vi "map_trap_switch.vi"() -> ()   [LabVIEW 2015]
panel:
  in  "KILL":bool
  in  "PAUSE":bool
  in  "RESUME":bool
  in  "QUIT":bool
  in  "up done":bool
  in  "z up":bool
  in  "Done":bool
  in  "z piastra 2":bool
  in  "z piastra":bool
  in  "y piastra":bool
  in  "x piastra":bool
  in  "goto y pos":bool
  in  "goto x pos":bool
  in  "Panello o piastre?":bool
  in  "End":bool
  in  "zero z - end":bool
  in  "zero x - end":bool
  in  "zero y - end":bool
  in  "goto z pos":bool
  in  "positioning done":bool
  out "output":string
  out "command":string
  in  "zero done":bool
  in  "zero z":bool
  in  "zero x":bool
  in  "zero y":bool
  # "Comandi di emergenza"
  # "Mappatura a trapezio \nper il pannello e le piastre"
  # "In alto: TRUE ---> Panello"
  # "In basso: FALSE ---> Piastre"
  # "Posiziono in zero"
  # "Vado sulla piastra \ne azzero"
  # "Alzo il comparatore"
  # "Vado in posizione"
  # "Ritorno a zero"
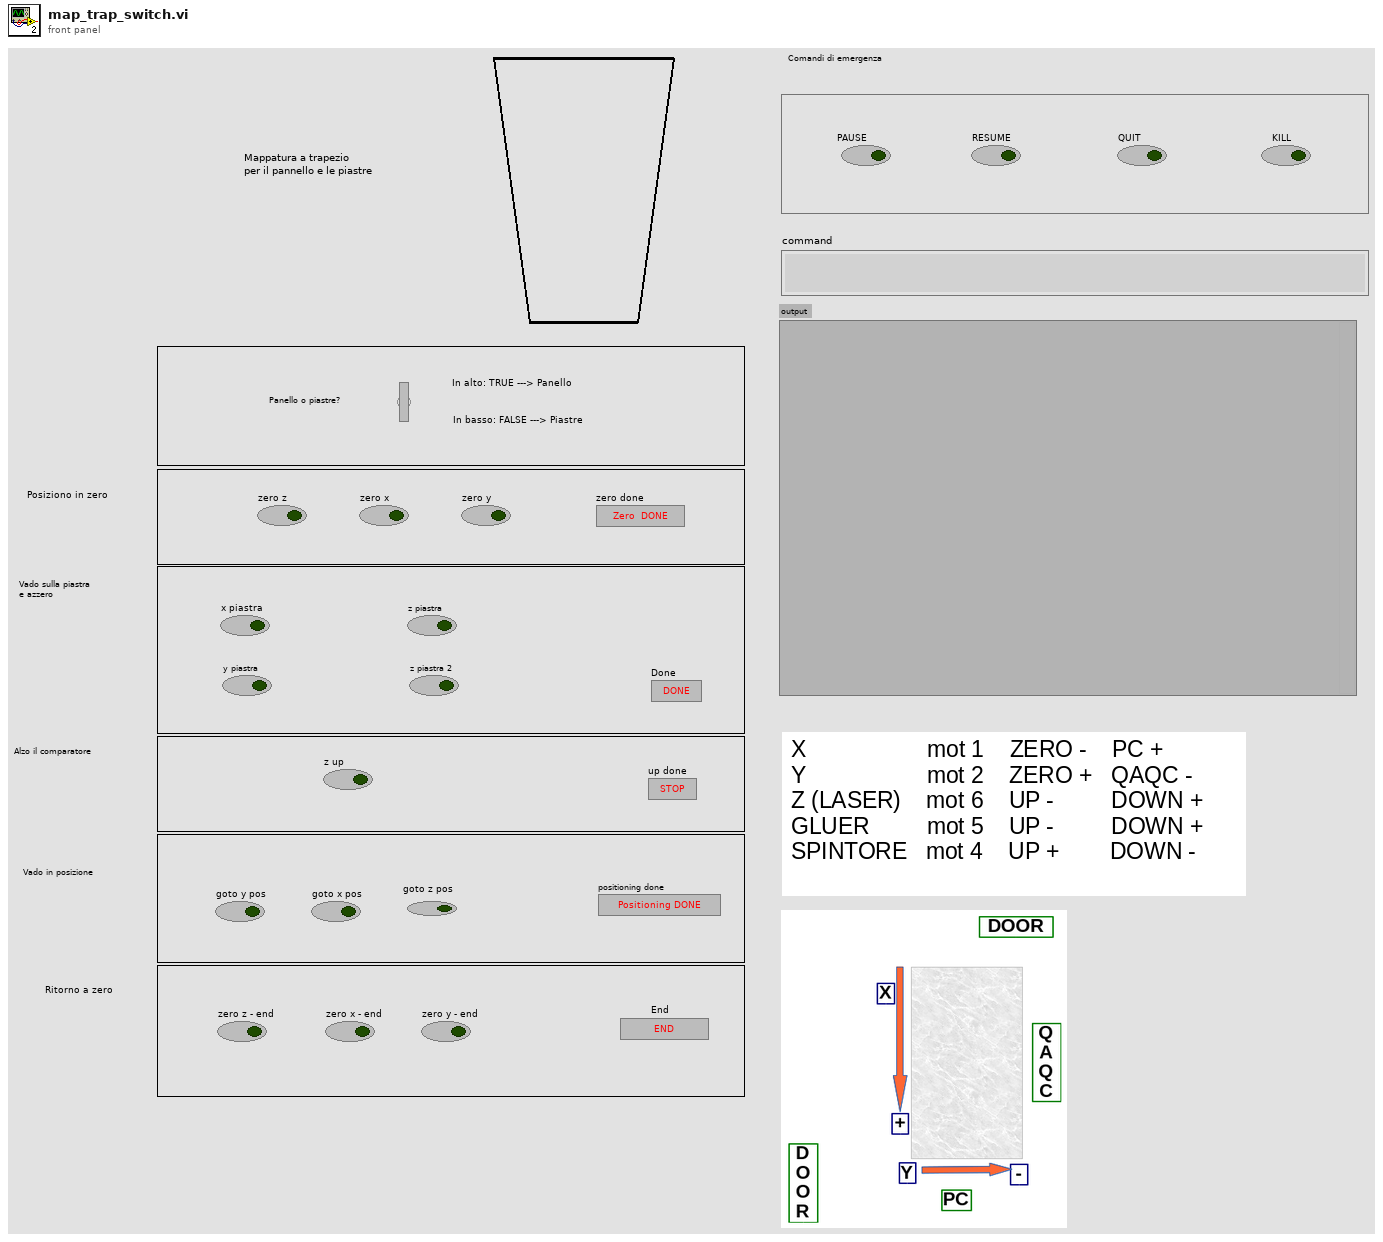
[diagram p1: front panel]
types:
  T1 = enum8{"Enabled", "Disabled", "Disabled and Grayed Out"}
  T2 = enum16{"open", "replace", "create", "open or create", "replace or create", "replace or create with confirmation"}
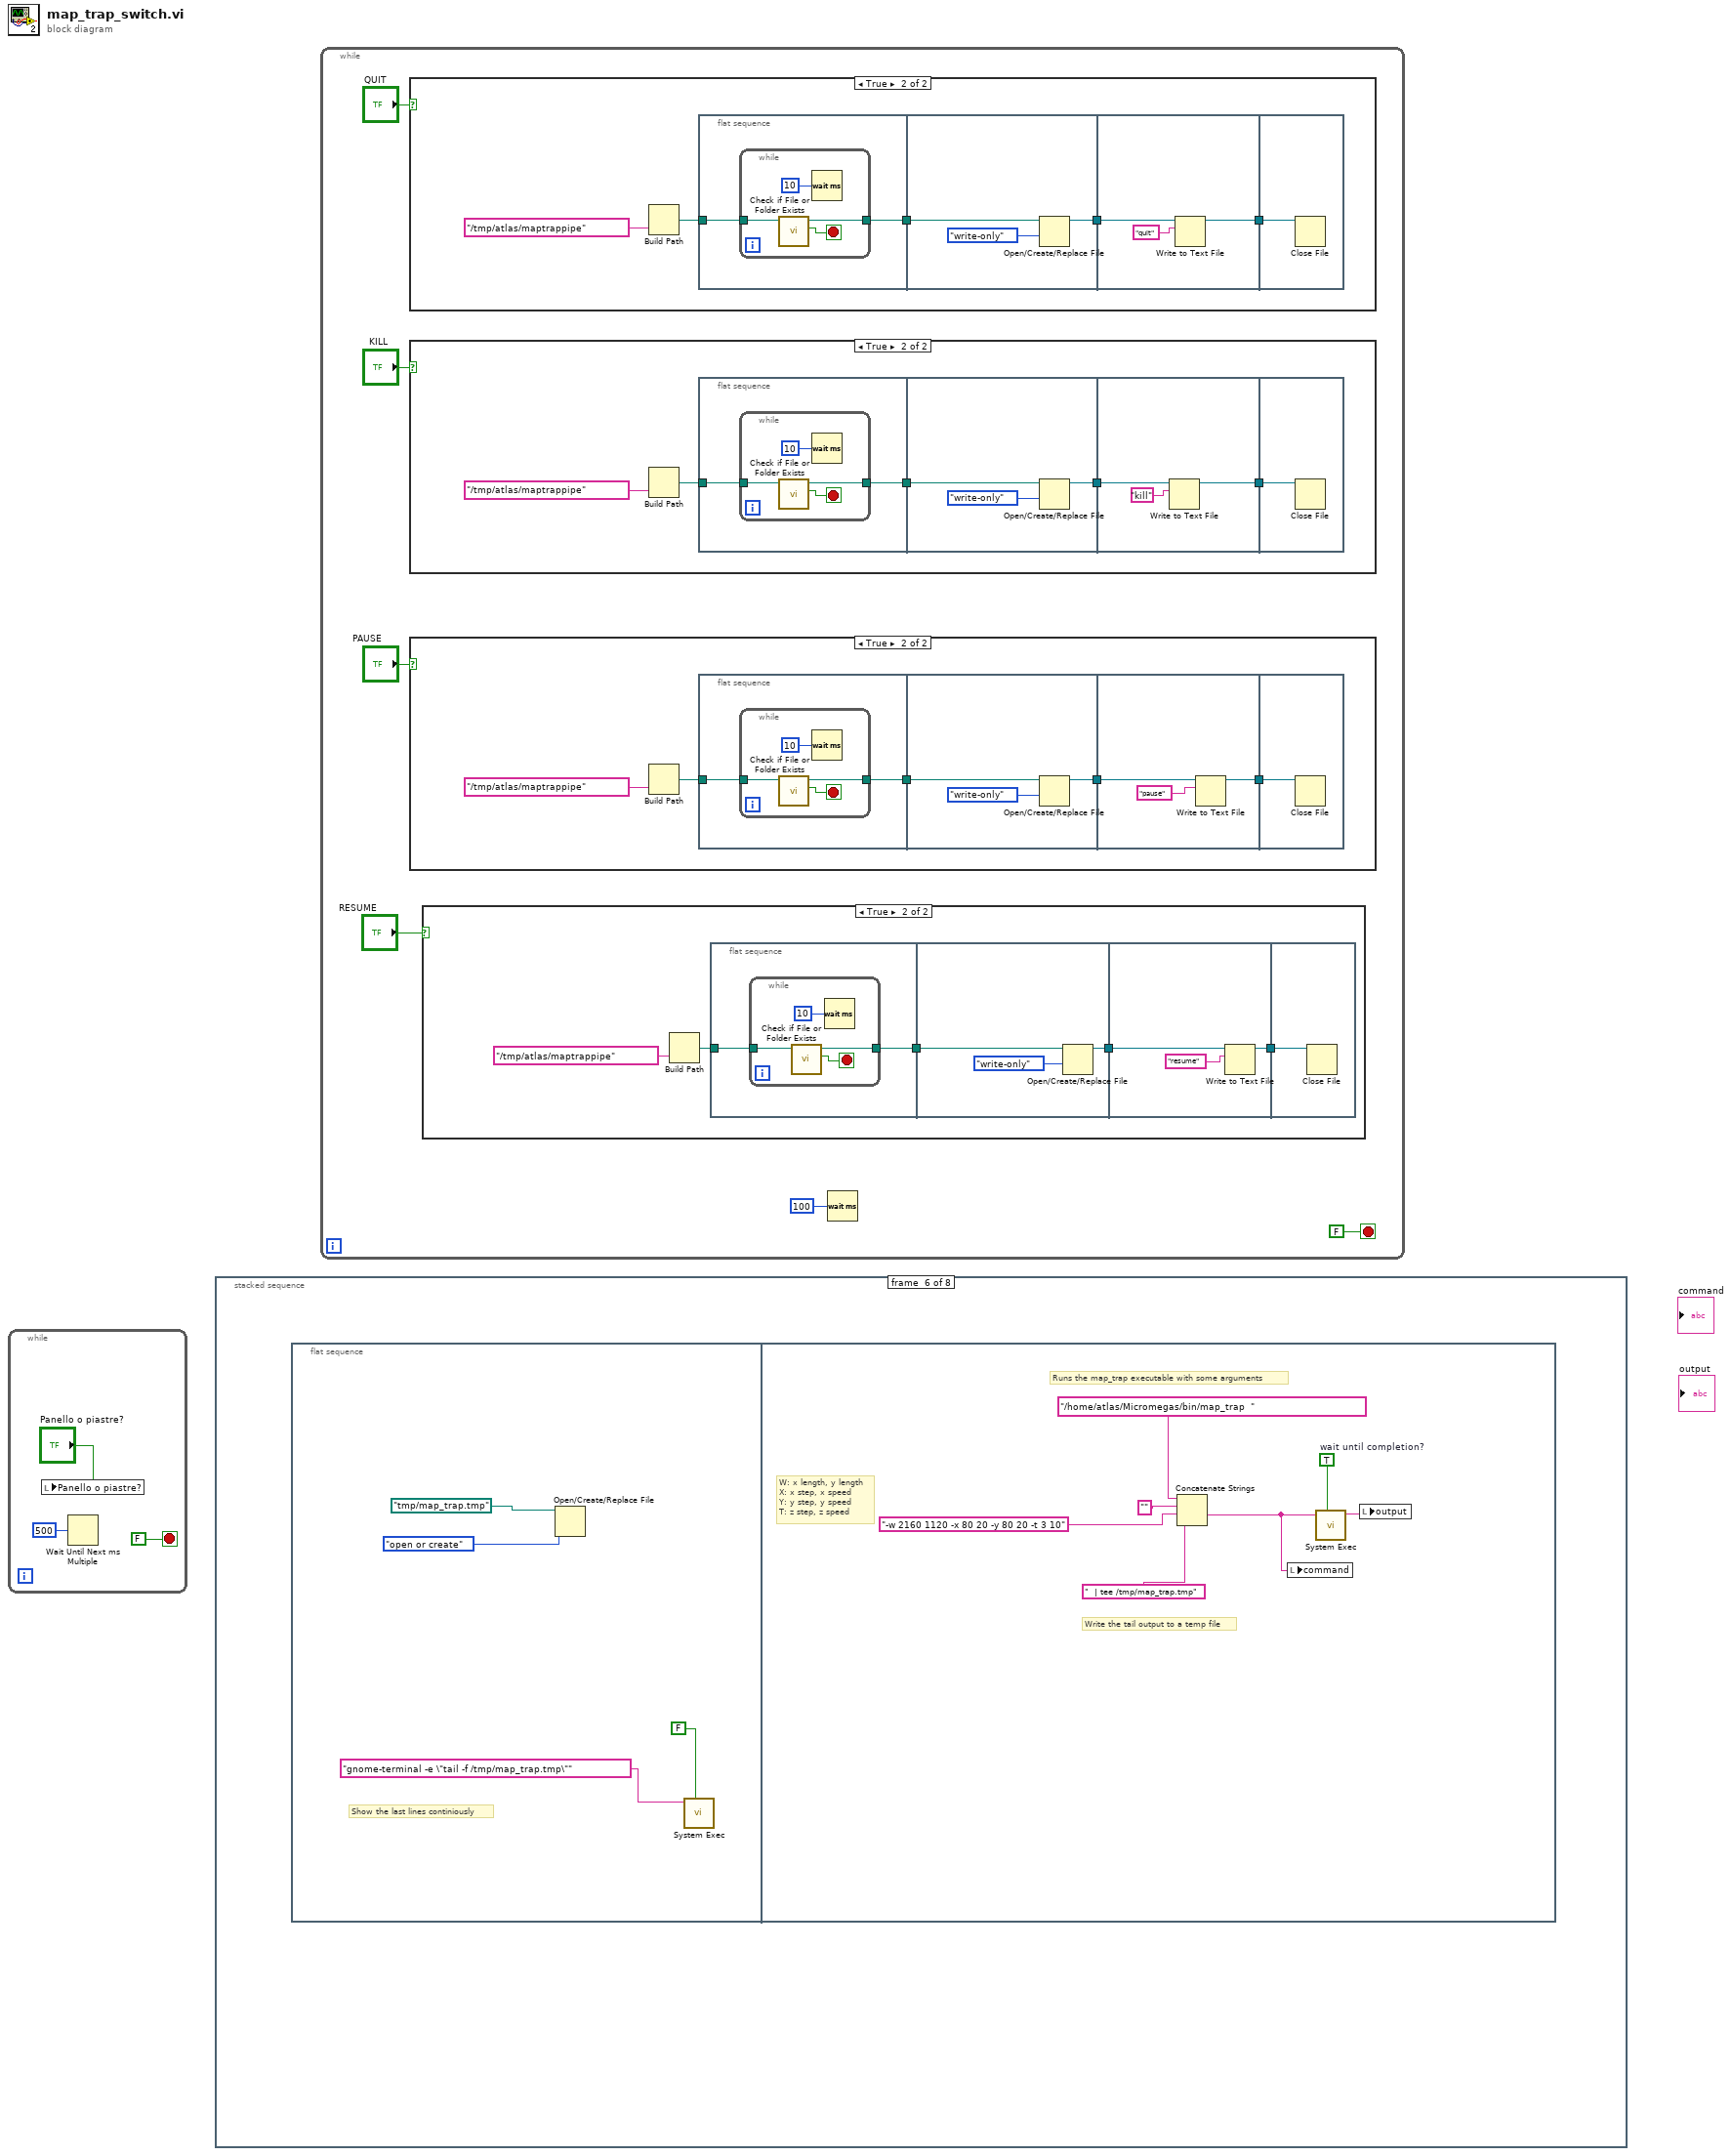
[diagram p0: block diagram]
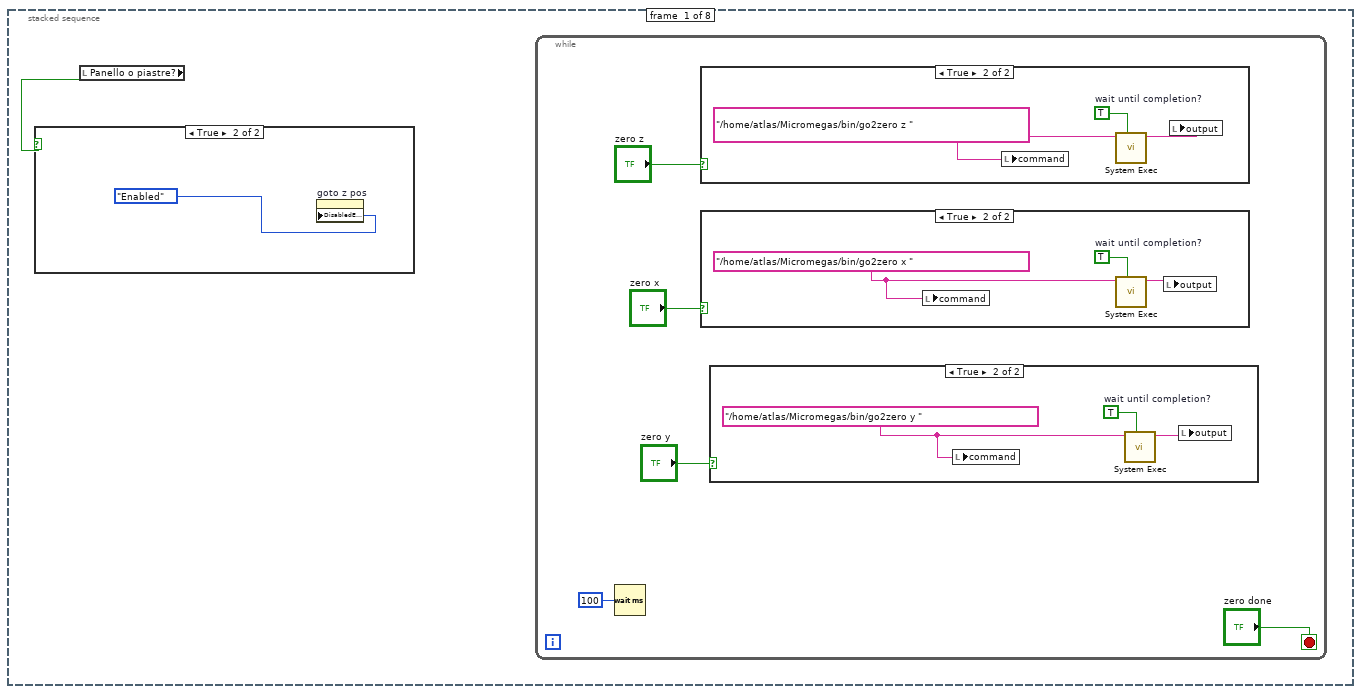
[diagram p6: hidden frame]
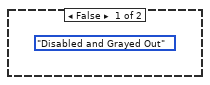
[diagram p7: hidden frame]
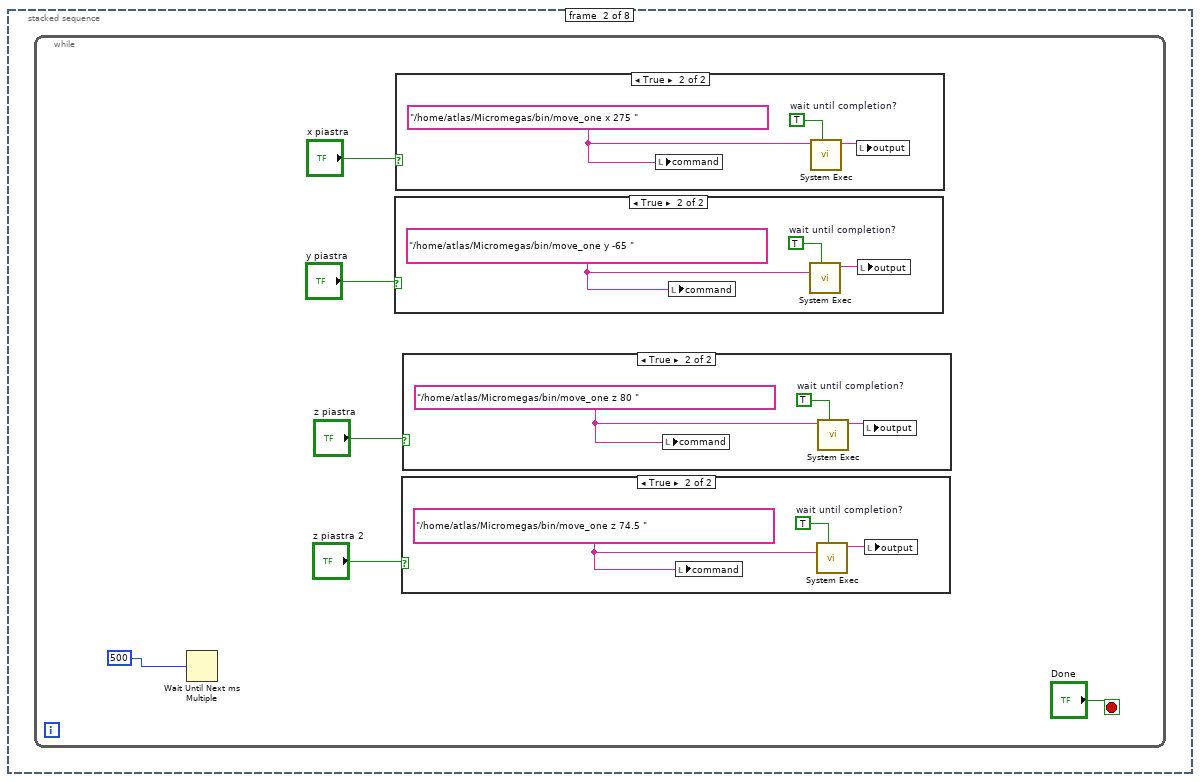
[diagram p11: hidden frame]
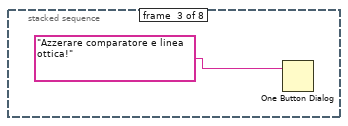
[diagram p16: hidden frame]
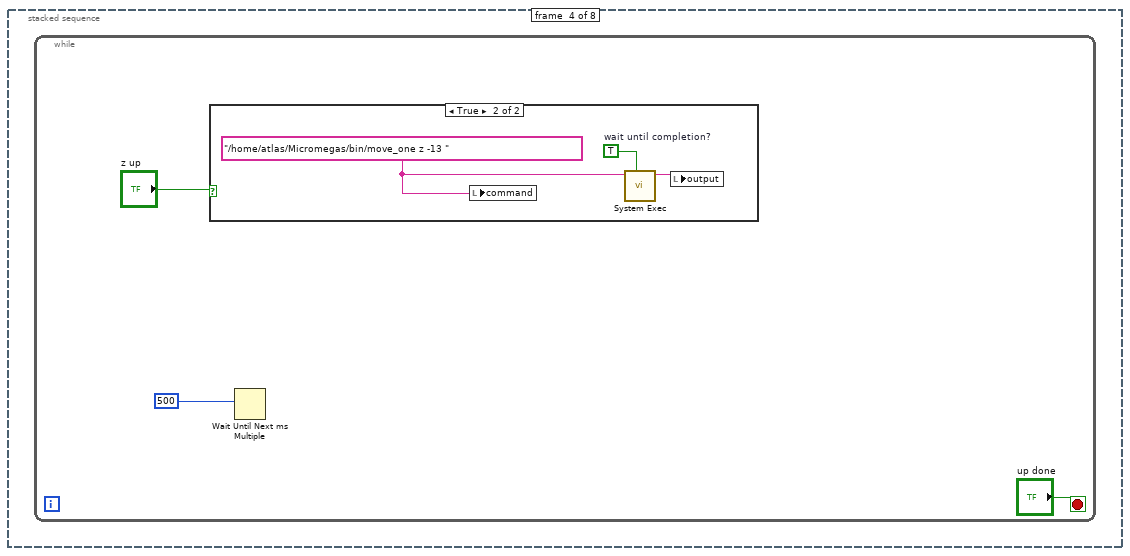
[diagram p17: hidden frame]
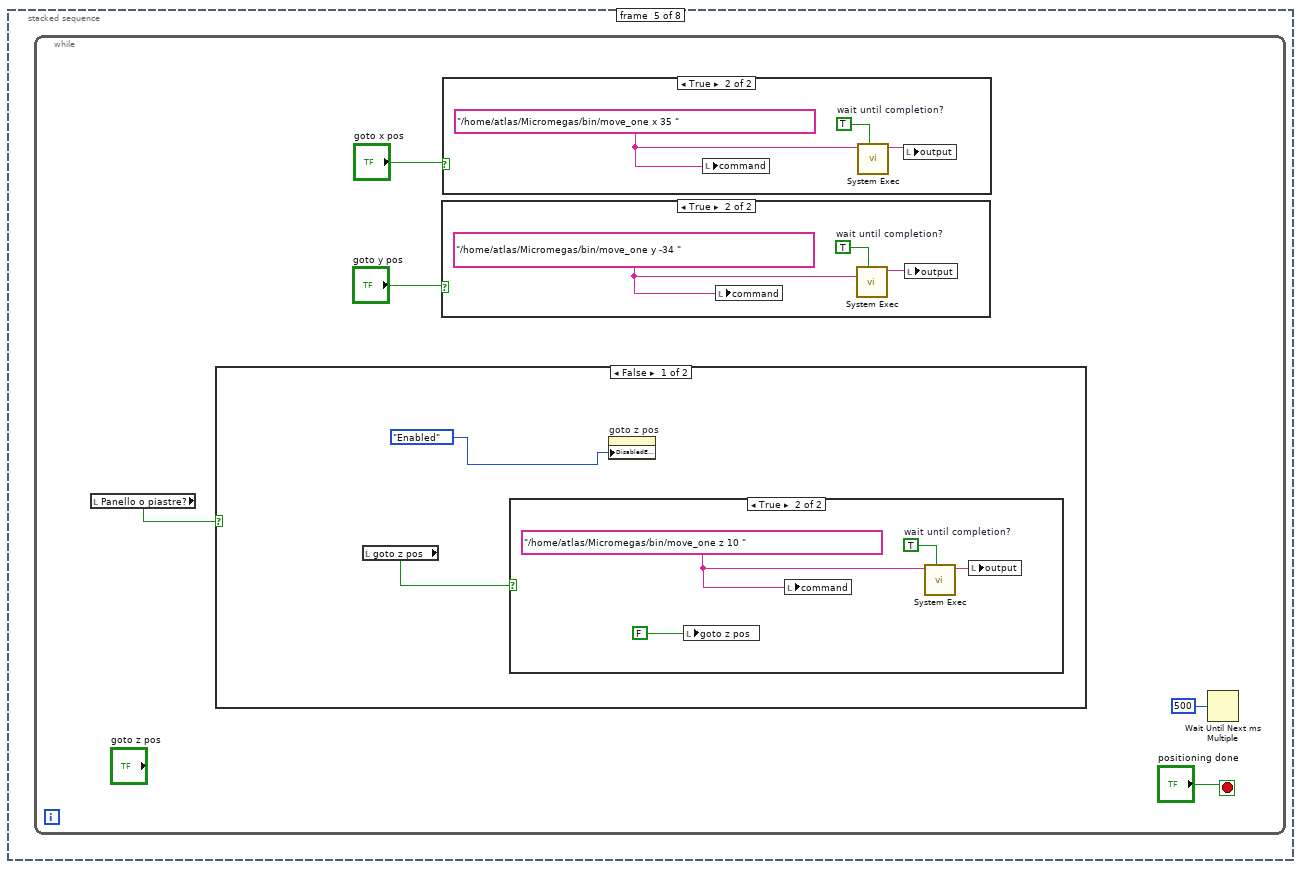
[diagram p19: hidden frame]
diagram:
  n1 = while {
    stop <- FALSE stop-if-true
    n2 = local write "Panello o piastre?"("Panello o piastre?") -> ()
    n3 = Wait Until Next ms Multiple(millisecond multiple=u32 500) -> ()  [unwired: 1 out]
  }
  n4 = stacked-sequence {
    frame #0 {
      n5 = local read "Panello o piastre?"() -> (w4:bool)
      n6 = case shown="True" w4 {
        frame False {
          (unwired) T1."Disabled and Grayed Out" ("Disabled")
        }
        frame True {
          n7 = property on="goto z pos" class="Bool (strict)"("DisabledEnum"=T1."Enabled" ("Disabled")) -> ()  [unwired: 2 in, 2 out]
        }
      }
      n8 = while {
        stop <- "zero done" stop-if-true
        n9 = Wait (ms)(milliseconds to wait=u32 100) -> ()  [unwired: 1 out]
        n10 = case shown="True" "zero z" {
          frame False {
          }
          frame True {
            w18 = "/home/atlas/Micromegas/bin/go2zero z " ("string")
            w19 = TRUE  # wait until completion?
            n11 = local write "command"(w18) -> ()
            n12 = call <vilib>:"System Exec.vi"("wait until completion? (T)"=w19, "command line"=w18) -> ("standard output"=w17:string)  [unwired: 6 in, 3 out]
            n13 = local write "output"(w17) -> ()
          }
        }
        n14 = case shown="True" "zero x" {
          frame False {
          }
          frame True {
            w15 = "/home/atlas/Micromegas/bin/go2zero x " ("string")
            w16 = TRUE  # wait until completion?
            n15 = local write "command"(w15) -> ()
            n16 = call <vilib>:"System Exec.vi"("wait until completion? (T)"=w16, "command line"=w15) -> ("standard output"=w14:string)  [unwired: 6 in, 3 out]
            n17 = local write "output"(w14) -> ()
          }
        }
        n18 = case shown="True" "zero y" {
          frame False {
          }
          frame True {
            w12 = "/home/atlas/Micromegas/bin/go2zero y " ("string")
            w13 = TRUE  # wait until completion?
            n19 = local write "command"(w12) -> ()
            n20 = call <vilib>:"System Exec.vi"("wait until completion? (T)"=w13, "command line"=w12) -> ("standard output"=w11:string)  [unwired: 6 in, 3 out]
            n21 = local write "output"(w11) -> ()
          }
        }
      }
    }
    frame #1 {
      n22 = while {
        stop <- "Done" stop-if-true
        n23 = Wait Until Next ms Multiple(millisecond multiple=u32 500 ("millisecond timer value")) -> ()  [unwired: 1 out]
        n24 = case shown="True" "y piastra" {
          frame False {
          }
          frame True {
            w32 = "/home/atlas/Micromegas/bin/move_one y -65 " ("string")
            w34 = TRUE  # wait until completion?
            n25 = local write "command"(w32) -> ()
            n26 = call <vilib>:"System Exec.vi"("wait until completion? (T)"=w34, "command line"=w32) -> ("standard output"=w33:string)  [unwired: 6 in, 3 out]
            n27 = local write "output"(w33) -> ()
          }
        }
        n28 = case shown="True" "x piastra" {
          frame False {
          }
          frame True {
            w35 = "/home/atlas/Micromegas/bin/move_one x 275 " ("string")
            w37 = TRUE  # wait until completion?
            n29 = local write "command"(w35) -> ()
            n30 = call <vilib>:"System Exec.vi"("wait until completion? (T)"=w37, "command line"=w35) -> ("standard output"=w36:string)  [unwired: 6 in, 3 out]
            n31 = local write "output"(w36) -> ()
          }
        }
        n32 = case shown="True" "z piastra 2" {
          frame False {
          }
          frame True {
            w26 = "/home/atlas/Micromegas/bin/move_one z 74.5 " ("string")
            w28 = TRUE  # wait until completion?
            n33 = local write "command"(w26) -> ()
            n34 = call <vilib>:"System Exec.vi"("wait until completion? (T)"=w28, "command line"=w26) -> ("standard output"=w27:string)  [unwired: 6 in, 3 out]
            n35 = local write "output"(w27) -> ()
          }
        }
        n36 = case shown="True" "z piastra" {
          frame False {
          }
          frame True {
            w29 = "/home/atlas/Micromegas/bin/move_one z 80 " ("string")
            w31 = TRUE  # wait until completion?
            n37 = local write "command"(w29) -> ()
            n38 = call <vilib>:"System Exec.vi"("wait until completion? (T)"=w31, "command line"=w29) -> ("standard output"=w30:string)  [unwired: 6 in, 3 out]
            n39 = local write "output"(w30) -> ()
          }
        }
      }
    }
    frame #2 {
      n40 = One Button Dialog(message="Azzerare comparatore e linea ottica!") -> ()  [unwired: 1 in, 1 out]
    }
    frame #3 {
      n41 = while {
        stop <- "up done" stop-if-true
        n42 = case shown="True" "z up" {
          frame False {
          }
          frame True {
            w42 = "/home/atlas/Micromegas/bin/move_one z -13 " ("string")
            w44 = TRUE  # wait until completion?
            n43 = local write "command"(w42) -> ()
            n44 = call <vilib>:"System Exec.vi"("wait until completion? (T)"=w44, "command line"=w42) -> ("standard output"=w43:string)  [unwired: 6 in, 3 out]
            n45 = local write "output"(w43) -> ()
          }
        }
        n46 = Wait Until Next ms Multiple(millisecond multiple=u32 500 ("millisecond timer value")) -> ()  [unwired: 1 out]
      }
    }
    frame #4 {
      n47 = while {
        stop <- "positioning done" stop-if-true
        n48 = local read "Panello o piastre?"() -> (w45:bool)
        n49 = case shown="False" w45 {
          frame False {
            n50 = local read "goto z pos"() -> (w51:bool)
            n51 = case shown="True" w51 {
              frame False {
              }
              frame True {
                w53 = "/home/atlas/Micromegas/bin/move_one z 10 " ("string")
                w55 = TRUE  # wait until completion?
                n52 = local write "goto z pos"(FALSE ("goto z pos")) -> ()
                n53 = local write "command"(w53) -> ()
                n54 = call <vilib>:"System Exec.vi"("wait until completion? (T)"=w55, "command line"=w53) -> ("standard output"=w54:string)  [unwired: 6 in, 3 out]
                n55 = local write "output"(w54) -> ()
              }
            }
            n56 = property on="goto z pos" class="Bool (strict)"("DisabledEnum"=T1."Enabled" ("Disabled")) -> ()  [unwired: 2 in, 2 out]
          }
          frame True {
            n57 = property on="goto z pos" class="Bool (strict)"("DisabledEnum"=T1."Disabled and Grayed Out" ("Disabled")) -> ()  [unwired: 2 in, 2 out]
          }
        }
        n58 = case shown="True" "goto y pos" {
          frame False {
          }
          frame True {
            w57 = "/home/atlas/Micromegas/bin/move_one y -34 " ("string")
            w59 = TRUE  # wait until completion?
            n59 = local write "command"(w57) -> ()
            n60 = call <vilib>:"System Exec.vi"("wait until completion? (T)"=w59, "command line"=w57) -> ("standard output"=w58:string)  [unwired: 6 in, 3 out]
            n61 = local write "output"(w58) -> ()
          }
        }
        n62 = case shown="True" "goto x pos" {
          frame False {
          }
          frame True {
            w60 = "/home/atlas/Micromegas/bin/move_one x 35 " ("string")
            w62 = TRUE  # wait until completion?
            n63 = local write "command"(w60) -> ()
            n64 = call <vilib>:"System Exec.vi"("wait until completion? (T)"=w62, "command line"=w60) -> ("standard output"=w61:string)  [unwired: 6 in, 3 out]
            n65 = local write "output"(w61) -> ()
          }
        }
        n66 = Wait Until Next ms Multiple(millisecond multiple=u32 500) -> ()  [unwired: 1 out]
      }
    }
    frame #5 {
      n67 = flat-sequence {
        frame #0 {
          # "Show the last lines continiously"
          n68 = Open/Create/Replace File(file path (use dialog)=path "/tmp/map_trap.tmp", operation (0:open)=T2."open or create") -> ()  [unwired: 4 in, 3 out]
          n69 = call <vilib>:"System Exec.vi"("wait until completion? (T)"=FALSE, "command line"="gnome-terminal -e \"tail -f /tmp/map_trap.tmp\"") -> ()  [unwired: 6 in, 4 out]
        }
        frame #1 {
          w73 = TRUE  # wait until completion?
          # "Write the tail output to a temp file"
          # "Runs the map_trap executable with some arguments"
          # "W: x length, y length\nX: x step, x speed\nY: y step, y speed\nT: z step, z speed"
          n70 = Concatenate Strings("/home/atlas/Micromegas/bin/map_trap  " ("string"), "" ("string"), "-w 2160 1120 -x 80 20 -y 80 20 -t 3 10" ("string"), "  | tee /tmp/map_trap.tmp" ("string")) -> (w68:string)
          n71 = local write "command"(w68) -> ()
          n72 = call <vilib>:"System Exec.vi"("wait until completion? (T)"=w73, "command line"=w68) -> ("standard output"=w67:string)  [unwired: 6 in, 3 out]
          n73 = local write "output"(w67) -> ()
        }
      }
    }
    frame #6 {
      n74 = while {
        stop <- "End" stop-if-true
        n75 = Wait (ms)(milliseconds to wait=u32 100) -> ()  [unwired: 1 out]
        n76 = case shown="True" "zero z - end" {
          frame False {
          }
          frame True {
            w86 = "/home/atlas/Micromegas/bin/go2zero z " ("string")
            w87 = TRUE  # wait until completion?
            n77 = local write "command"(w86) -> ()
            n78 = call <vilib>:"System Exec.vi"("wait until completion? (T)"=w87, "command line"=w86) -> ("standard output"=w85:string)  [unwired: 6 in, 3 out]
            n79 = local write "output"(w85) -> ()
          }
        }
        n80 = case shown="True" "zero x - end" {
          frame False {
          }
          frame True {
            w83 = "/home/atlas/Micromegas/bin/go2zero x " ("string")
            w84 = TRUE  # wait until completion?
            n81 = local write "command"(w83) -> ()
            n82 = call <vilib>:"System Exec.vi"("wait until completion? (T)"=w84, "command line"=w83) -> ("standard output"=w82:string)  [unwired: 6 in, 3 out]
            n83 = local write "output"(w82) -> ()
          }
        }
        n84 = case shown="True" "zero y - end" {
          frame False {
          }
          frame True {
            w80 = "/home/atlas/Micromegas/bin/go2zero y " ("string")
            w81 = TRUE  # wait until completion?
            n85 = local write "command"(w80) -> ()
            n86 = call <vilib>:"System Exec.vi"("wait until completion? (T)"=w81, "command line"=w80) -> ("standard output"=w79:string)  [unwired: 6 in, 3 out]
            n87 = local write "output"(w79) -> ()
          }
        }
      }
    }
    frame #7 {
      n88 = One Button Dialog(message="Per comodita`, rinominare il file (non verra` comunque sovrascritto)") -> ()  [unwired: 1 in, 1 out]
    }
  }
  n89 = while {
    stop <- FALSE stop-if-true
    n90 = case shown="True" "QUIT" {
      frame False {
      }
      frame True {
        n91 = Build Path(name or relative path="/tmp/atlas/maptrappipe" ("string")) -> (appended path=w149:path)  [unwired: 1 in]
        n92 = flat-sequence {
          tunnel: [w155] -> w153
          tunnel: w149 -> [w154]
          tunnel: w153 -> [w162]
          tunnel: [w160] -> w152
          tunnel: w152 -> [w165]
          tunnel: [w164] -> w151
          tunnel: w151 -> [w166]
          frame #0 {
            n93 = while {
              tunnel: [w157] -> w155
              tunnel: w154 -> [w156]
              stop <- w158 stop-if-true
              n94 = call <vilib>:"Check if File or Folder Exists.vi"("path"=w156) -> ("file or folder exists?"=w158:bool, "dup path"=w157:path)  [unwired: 8 in, 1 out]
              n95 = Wait (ms)(milliseconds to wait=u32 10) -> ()  [unwired: 1 out]
            }
          }
          frame #1 {
            n96 = Open/Create/Replace File(file path (use dialog)=w162, access (0:read/write)=enum16{"read/write", "read-only", "write-only"}."write-only") -> (refnum out=w160:refnum<file>)  [unwired: 4 in, 2 out]
          }
          frame #2 {
            n97 = Write to Text File(file (use dialog)=w165, text="quit") -> (refnum out=w164:refnum<file>)  [unwired: 2 in, 2 out]
          }
          frame #3 {
            n98 = Close File(refnum=w166) -> ()  [unwired: 1 in, 2 out]
          }
        }
      }
    }
    n99 = case shown="True" "KILL" {
      frame False {
      }
      frame True {
        n100 = Build Path(name or relative path="/tmp/atlas/maptrappipe" ("string")) -> (appended path=w113:path)  [unwired: 1 in]
        n101 = flat-sequence {
          tunnel: [w119] -> w117
          tunnel: w113 -> [w118]
          tunnel: w117 -> [w126]
          tunnel: [w124] -> w116
          tunnel: w116 -> [w129]
          tunnel: [w128] -> w115
          tunnel: w115 -> [w130]
          frame #0 {
            n102 = while {
              tunnel: [w121] -> w119
              tunnel: w118 -> [w120]
              stop <- w122 stop-if-true
              n103 = call <vilib>:"Check if File or Folder Exists.vi"("path"=w120) -> ("file or folder exists?"=w122:bool, "dup path"=w121:path)  [unwired: 8 in, 1 out]
              n104 = Wait (ms)(milliseconds to wait=u32 10) -> ()  [unwired: 1 out]
            }
          }
          frame #1 {
            n105 = Open/Create/Replace File(file path (use dialog)=w126, access (0:read/write)=enum16{"read/write", "read-only", "write-only"}."write-only") -> (refnum out=w124:refnum<file>)  [unwired: 4 in, 2 out]
          }
          frame #2 {
            n106 = Write to Text File(file (use dialog)=w129, text="kill") -> (refnum out=w128:refnum<file>)  [unwired: 2 in, 2 out]
          }
          frame #3 {
            n107 = Close File(refnum=w130) -> ()  [unwired: 1 in, 2 out]
          }
        }
      }
    }
    n108 = case shown="True" "PAUSE" {
      frame False {
      }
      frame True {
        n109 = Build Path(name or relative path="/tmp/atlas/maptrappipe" ("string")) -> (appended path=w95:path)  [unwired: 1 in]
        n110 = flat-sequence {
          tunnel: [w101] -> w99
          tunnel: w95 -> [w100]
          tunnel: w99 -> [w108]
          tunnel: [w106] -> w98
          tunnel: w98 -> [w111]
          tunnel: [w110] -> w97
          tunnel: w97 -> [w112]
          frame #0 {
            n111 = while {
              tunnel: [w103] -> w101
              tunnel: w100 -> [w102]
              stop <- w104 stop-if-true
              n112 = call <vilib>:"Check if File or Folder Exists.vi"("path"=w102) -> ("file or folder exists?"=w104:bool, "dup path"=w103:path)  [unwired: 8 in, 1 out]
              n113 = Wait (ms)(milliseconds to wait=u32 10) -> ()  [unwired: 1 out]
            }
          }
          frame #1 {
            n114 = Open/Create/Replace File(file path (use dialog)=w108, access (0:read/write)=enum16{"read/write", "read-only", "write-only"}."write-only") -> (refnum out=w106:refnum<file>)  [unwired: 4 in, 2 out]
          }
          frame #2 {
            n115 = Write to Text File(file (use dialog)=w111, text="pause") -> (refnum out=w110:refnum<file>)  [unwired: 2 in, 2 out]
          }
          frame #3 {
            n116 = Close File(refnum=w112) -> ()  [unwired: 1 in, 2 out]
          }
        }
      }
    }
    n117 = case shown="True" "RESUME" {
      frame False {
      }
      frame True {
        n118 = Build Path(name or relative path="/tmp/atlas/maptrappipe" ("string")) -> (appended path=w131:path)  [unwired: 1 in]
        n119 = flat-sequence {
          tunnel: [w137] -> w135
          tunnel: w131 -> [w136]
          tunnel: w135 -> [w144]
          tunnel: [w142] -> w134
          tunnel: w134 -> [w147]
          tunnel: [w146] -> w133
          tunnel: w133 -> [w148]
          frame #0 {
            n120 = while {
              tunnel: [w139] -> w137
              tunnel: w136 -> [w138]
              stop <- w140 stop-if-true
              n121 = call <vilib>:"Check if File or Folder Exists.vi"("path"=w138) -> ("file or folder exists?"=w140:bool, "dup path"=w139:path)  [unwired: 8 in, 1 out]
              n122 = Wait (ms)(milliseconds to wait=u32 10) -> ()  [unwired: 1 out]
            }
          }
          frame #1 {
            n123 = Open/Create/Replace File(file path (use dialog)=w144, access (0:read/write)=enum16{"read/write", "read-only", "write-only"}."write-only") -> (refnum out=w142:refnum<file>)  [unwired: 4 in, 2 out]
          }
          frame #2 {
            n124 = Write to Text File(file (use dialog)=w147, text="resume") -> (refnum out=w146:refnum<file>)  [unwired: 2 in, 2 out]
          }
          frame #3 {
            n125 = Close File(refnum=w148) -> ()  [unwired: 1 in, 2 out]
          }
        }
      }
    }
    n126 = Wait (ms)(milliseconds to wait=100) -> ()  [unwired: 1 out]
  }
